vi "To XML - Invalid character in Classname - XML does not contain invalid character.vi"() -> ()   [LabVIEW 2013, in "JUnit XML Tests.lvlib" / "Test Case.lvlib"]
uses:
  Test Case.lvlib
  JUnit XML/Test Case/Test Case.lvclass
  <vilib>/xml/Close Reference(Node).vi
  <vilib>/addons/_JKI Toolkits/Caraya/classes/Assert/Assert Equal Value_Variant.vi
  <vilib>/addons/_JKI Toolkits/Caraya/classes/Test/Test.lvclass
  <vilib>/addons/_JKI Toolkits/Caraya/classes/Assert/Assert.lvclass
  <resource>/objmgr/DOMUserDefRef.rc
  <vilib>/xml/NI_XML.lvlib
panel:
  out "error out":errorcluster
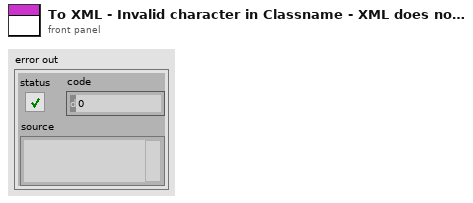
[diagram p1: front panel]
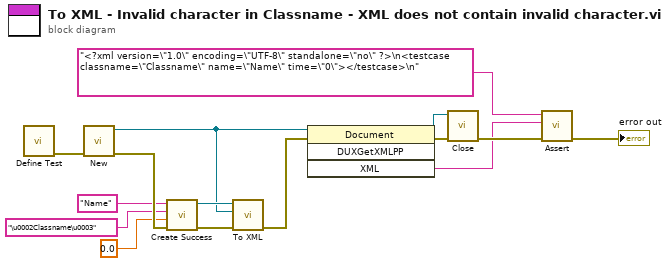
[diagram p0: block diagram]
diagram:
  n1 = call <vilib>:"Define Test.vi"() -> ("error out"=w15:errorcluster)  [unwired: 10 in, 1 out]
  n2 = call <vilib>:"New.vi"("error in (no error)"=w15) -> ("error out"=w12:errorcluster, "DOM document out"=w2:refnum<k20>)  [unwired: 7 in]
  n3 = call "Create Success.vi"("error in (no error)"=w12, "Time"=0.0, "Classname"="\u0002Classname\u0003", "Name"="Name") -> ("error out"=w13:errorcluster, "Test Case"=w14:refnum<class "Test Case.lvclass">)  [unwired: 6 in]
  n4 = call-dynamic "To XML.vi"("error in (no error)"=w13, "Parent"=w2, "Test Case in"=w14) -> ("error out"=w1:errorcluster)  [unwired: 8 in]
  n5 = invoke class="Document" method="DUXGetXMLPP"(reference=w2, error in=w1) -> (reference out=w10:refnum<k20>, error out=w11:errorcluster, "XML"=w8:string)  [unwired: 2 in, 1 out]
  n6 = call-poly <vilib>:"Close.vi"("error in (no error)"=w11, "node"=w10) -> ("error out"=w9:errorcluster)  [unwired: 7 in]
  n7 = call-poly <vilib>:"Assert.vi"("error in (no error)"=w9, "Actual"=w8, "Expected"="<?xml version=\"1.0\" encoding=\"UTF-8\" standalone=\"no\" ?>\n<testcase classname=\"Classname\" name=\"Name\" time=\"0\"></testcase>\n") -> ("error out"=→"error out":errorcluster)  [unwired: 7 in, 1 out]
